vi "Apollo_global_variable.vi"(4 "2D array input":dbl[][](array[numeric]) format="%0.2f", 5 "Engineering num precision default is  (6)":i16, 6 "Global variable types":T1(ring), 7 "Engineering number input":dbl, 8 "variable name":string, 9 "1D Array input":dbl[](array[numeric]) format="%0.2f", 10 "String input":string, 11 "Single decimal number":i32) -> ()   [LabVIEW 2010]
uses:
  <vilib>/Utility/file.llb/Write To Spreadsheet File (DBL).vi
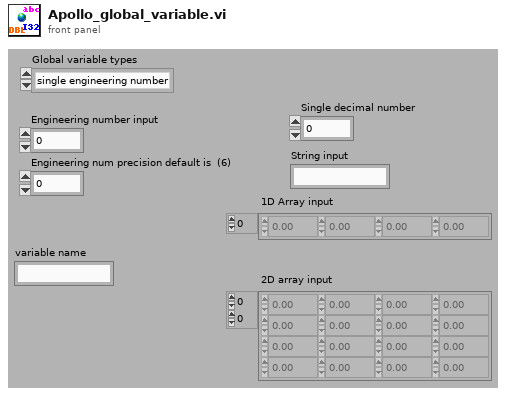
[diagram p1: front panel]
types:
  T1 = enum16{"single engineering number", "single decimal number", "1D Array input", "string", "2D array input"}
  T2 = enum16{"open", "replace", "create", "open or create", "replace or create", "replace or create with confirmation"}
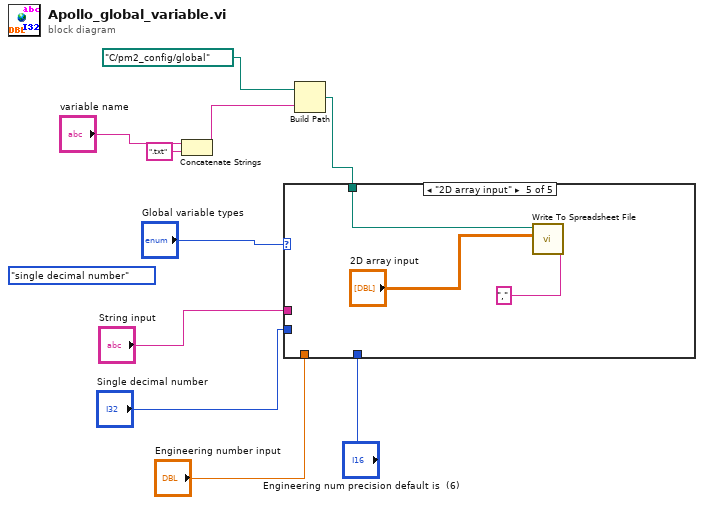
[diagram p0: block diagram]
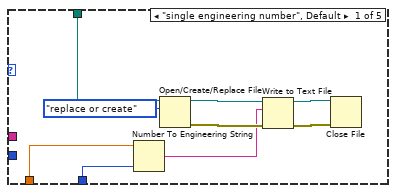
[diagram p2: hidden frame]
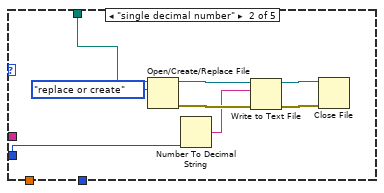
[diagram p3: hidden frame]
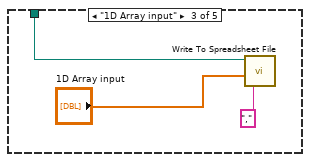
[diagram p4: hidden frame]
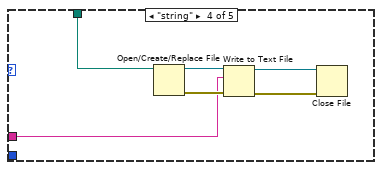
[diagram p5: hidden frame]
diagram:
  (unwired) T1."single decimal number"
  n1 = Concatenate Strings("variable name", ".txt" ("string")) -> (w9:string)
  n2 = Build Path(base path=path "C:/pm2_config/global", name or relative path=w9) -> (appended path=w8:path)
  n3 = case shown="\"2D array input\"" "Global variable types" {
    tunnel: w8 -> [w18 w21 w30 w32 w38]
    tunnel: "String input" -> [_ _ _ w31 _]
    tunnel: "Single decimal number" -> [_ w20 _ _ _]
    tunnel: "Engineering num precision default is  (6)" -> [w12 _ _ _ _]
    tunnel: "Engineering number input" -> [w11 _ _ _ _]
    frame "single engineering number", Default {
      n4 = Number To Engineering String(2:w12, 4:w11) -> (0:w13:string)  [unwired: 2 in]
      n5 = Open/Create/Replace File(file path (use dialog)=w18, operation (0:open)=T2."replace or create") -> (refnum out=w17:refnum<file>, error out=w19:errorcluster)  [unwired: 4 in, 1 out]
      n6 = Write to Text File(file (use dialog)=w17, text=w13, error in=w19) -> (refnum out=w16:refnum<file>, error out=w15:errorcluster)  [unwired: 1 in, 1 out]
      n7 = Close File(refnum=w16, error in=w15) -> ()  [unwired: 2 out]
    }
    frame "single decimal number" {
      n8 = Open/Create/Replace File(file path (use dialog)=w21, operation (0:open)=T2."replace or create") -> (refnum out=w26:refnum<file>, error out=w27:errorcluster)  [unwired: 4 in, 1 out]
      n9 = Number To Decimal String(number=w20) -> (decimal integer string=w23:string)  [unwired: 1 in]
      n10 = Write to Text File(file (use dialog)=w26, text=w23, error in=w27) -> (refnum out=w25:refnum<file>, error out=w24:errorcluster)  [unwired: 1 in, 1 out]
      n11 = Close File(refnum=w25, error in=w24) -> ()  [unwired: 2 out]
    }
    frame "1D Array input" {
      n12 = call-poly <vilib>:"Write To Spreadsheet File.vi"("delimiter (\\t)"="," ("delimiter (\\t)"), "1D data"="1D Array input", "file path (dialog if empty)"=w30) -> ()  [unwired: 5 in, 1 out]
    }
    frame "string" {
      n13 = Open/Create/Replace File(file path (use dialog)=w32) -> (refnum out=w36:refnum<file>, error out=w34:errorcluster)  [unwired: 5 in, 1 out]
      n14 = Write to Text File(file (use dialog)=w36, text=w31, error in=w34) -> (refnum out=w35:refnum<file>, error out=w33:errorcluster)  [unwired: 1 in, 1 out]
      n15 = Close File(refnum=w35, error in=w33) -> ()  [unwired: 2 out]
    }
    frame "2D array input" {
      n16 = call-poly <vilib>:"Write To Spreadsheet File.vi"("delimiter (\\t)"="," ("delimiter (\\t)"), "2D data"="2D array input", "file path (dialog if empty)"=w38) -> ()  [unwired: 5 in, 1 out]
    }
  }
